vi "Control Panel.vi"(8 "error in (no error)":errorcluster, 11 "Fake Function Generator in":refnum<class "Function Generator.lvclass">) -> (0 "error out":errorcluster, 3 "Fake Function Generator out":refnum<class "Function Generator.lvclass">)   [LabVIEW 2009, in "Function Generator.lvclass"]
doc: "(Dynamic) A user-level application that simulates the physical front panel of the Instrument. Provide the user with buttons to manually control features of the instrument, and provide indicators of its current state."
uses:
  Function Generator.lvclass
  Tektronix AFG 3000 Series/controls.llb/Channel.ctl
  Tektronix AFG 3000 Series/controls.llb/Waveform Shape.ctl
  Tektronix AFG 3000 Series/controls.llb/Sweep Spacing.ctl
  Function Generator.lvclass/Function Generator.ctl
  Math Operations/To Start and Stop (bare).vi
  Math Operations/To Center and Span (frequency).vi
  Tektronix AFG 3000 Series/controls.llb/Voltage.ctl
  Tektronix AFG 3000 Series/controls.llb/Frequency Mode.ctl
  Tektronix AFG 3000 Series/controls.llb/Sweep Time Parameter.ctl
  Tektronix AFG 3000 Series/controls.llb/Sweep Frequency.ctl
  Math Operations/To Center and Span (bare).vi
  Math Operations/To Start and Stop (frequency).vi
  Tektronix AFG 3000 Series/Tektronix AFG 3000 Series.lvlib
  Utility Classes/Scannable/Scannable.lvclass
panel:
  in  "Ch2 on/off":bool
  in  "Ch1 on/off":bool
  out "Ready when blinking":bool
  in  "Set":bool
  in  "Read to control":bool
  in  "Read":bool
  in  "Copy actual to set":bool
  in  "Populate fields with member data":bool
  out "Start Freq.":dbl[unit]
  out "Stop Freq.":dbl[unit]
  out "Freq. Span":dbl[unit]
  out "Center Freq.":dbl[unit]
  out "Offset":dbl[unit]
  out "Amplitude":dbl[unit]
  out "High":dbl[unit]
  out "Low":dbl[unit]
  out "FM Source":u16(ring) items=["Internal", "External"]
  out "FM Modulation Waveform":u16(ring) items=["Sine", "Square", "Triangle", "Ramp", "Down Ramp", "Noise", "User 1", "User 2", "User 3", "User 4", "EMEMory", "EFILe"]
  out "FM Modulation Freq.":dbl[unit]=100.0
  out "FM Peak Deviation":dbl[unit]=100.0
  in  "FM Peak Deviation Set":dbl[unit]=100.0
  in  "FM Modulation Freq Set":dbl[unit]=100.0
  in  "FM Modulation Waveform Set":u16(ring) items=["Sine", "Square", "Triangle", "Ramp", "Down Ramp", "Noise", "User 1", "User 2", "User 3", "User 4", "EMEMory", "EFILe"]
  in  "FM Source Set":u16(ring) items=["Internal", "External"]
  out "AM Modulation Freq.":dbl[unit]=1000.0
  out "AM Modulation Waveform":u16(ring) items=["Sine", "Square", "Triangle", "Ramp", "Down Ramp", "Noise"]
  out "AM Source":u16(ring) items=["Internal", "External"]
  out "AM Modulation Depth":dbl
  in  "AM Modulation Depth Set":dbl
  in  "AM Modulation Freq. Set":dbl[unit]=1000.0
  in  "AM Modulation Waveform Set":u16(ring) items=["Sine", "Square", "Triangle", "Ramp", "Down Ramp", "Noise"]
  in  "AM Source Set":u16(ring) items=["Internal", "External"]
  out "Return Time":dbl[unit]
  out "Hold Time":dbl[unit]
  out "Sweep Time":dbl[unit]
  in  "Return Time Set":dbl[unit]
  in  "Hold Time Set":dbl[unit]
  in  "Sweep Time Set":dbl[unit] caption="Sweep time"
  out "Sweep Spacing":T1 items=["linear", "log"]
  in  "Sweep Spacing Set":T1 items=["linear", "log"]
  in  "Stop Freq. Set":dbl[unit]
  in  "Start Freq. Set":dbl[unit]
  out "Burst Mode":u16(ring)=1 items=["Triggered", "Gated"]
  out "Burst Count":i32=5
  in  "Burst Count Set":i32=5
  in  "Burst Mode Set":u16(ring)=1 items=["Triggered", "Gated"]
  out "Run Mode":u16(ring) items=["Continuous", "AM", "FM", "PM", "FSK", "PWM", "Sweep", "Burst"]
  in  "Run Mode Set":u16(ring) items=["Continuous", "AM", "FM", "PM", "FSK", "PWM", "Sweep", "Burst"]
  out "Trailing Edge Time":dbl[unit]
  out "Leading Edge Time":dbl[unit]
  out "Duty Cycle (%)":dbl
  in  "Duty Cycle Set (%)":dbl=50.0
  in  "Trailing Edge Time Set":dbl[unit]=5e-09 format="%#.6g"
  in  "Leading Edge Time Set":dbl[unit]=5e-09 format="%#.6g"
  out "Ramp Symm. (%)":dbl
  in  "Ramp Symm. Set (%)":dbl=50.0 min=0.0 max=100.0 step=1.0 format="%.2f"
  in  "Freq. Span Set":dbl[unit]
  in  "Center Freq. Set":dbl[unit]
  in  "Low Set":dbl[unit]
  in  "High Set":dbl[unit]
  in  "Amplitude Set":dbl[unit]
  in  "Offset Set":dbl[unit]
  in  "Exit":bool
  out "Waveform Shape":T2 items=["Sinusoid", "Square", "Pulse", "Ramp", "PRNoise", "DC", "SINC", "Gaussian", "Lorentz", "ERise", "EDecay", "Haversine", "User 1", "User 2", "User 3", "User 4", "EMemory", "EFile"]
  in  "Waveform Shape Set":T2 items=["Sinusoid", "Square", "Pulse", "Ramp", "PRNoise", "DC", "SINC", "Gaussian", "Lorentz", "ERise", "EDecay", "Haversine", "User 1", "User 2", "User 3", "User 4", "EMemory", "EFile"]
  out "Phase":dbl[unit]
  in  "Phase Set":dbl[unit]
  out "Frequency":dbl[unit]
  in  "Frequency Set":dbl[unit]
  in  "Channel":T3 items=["Channel 1", "Channel 2"]
  # "Tektronix AFG252 Function Generator Control Panel"
  # "VOLTAGE SETTINGS"
  # "SWEEP MODE SETTINGS"
  # "AM SETTINGS"
  # "GENERAL SETTINGS"
  # "RAMP SETTINGS"
  # "FM SETTINGS"
  # "Note: the program only sets\nthe values that are appropriate\nfor the run mode you select. I.e.,\nit won't set the FM settings if you\nselect \"Burst Mode\" here."
  # "PULSE SETTINGS"
  # "BURST MODE SETTINGS"
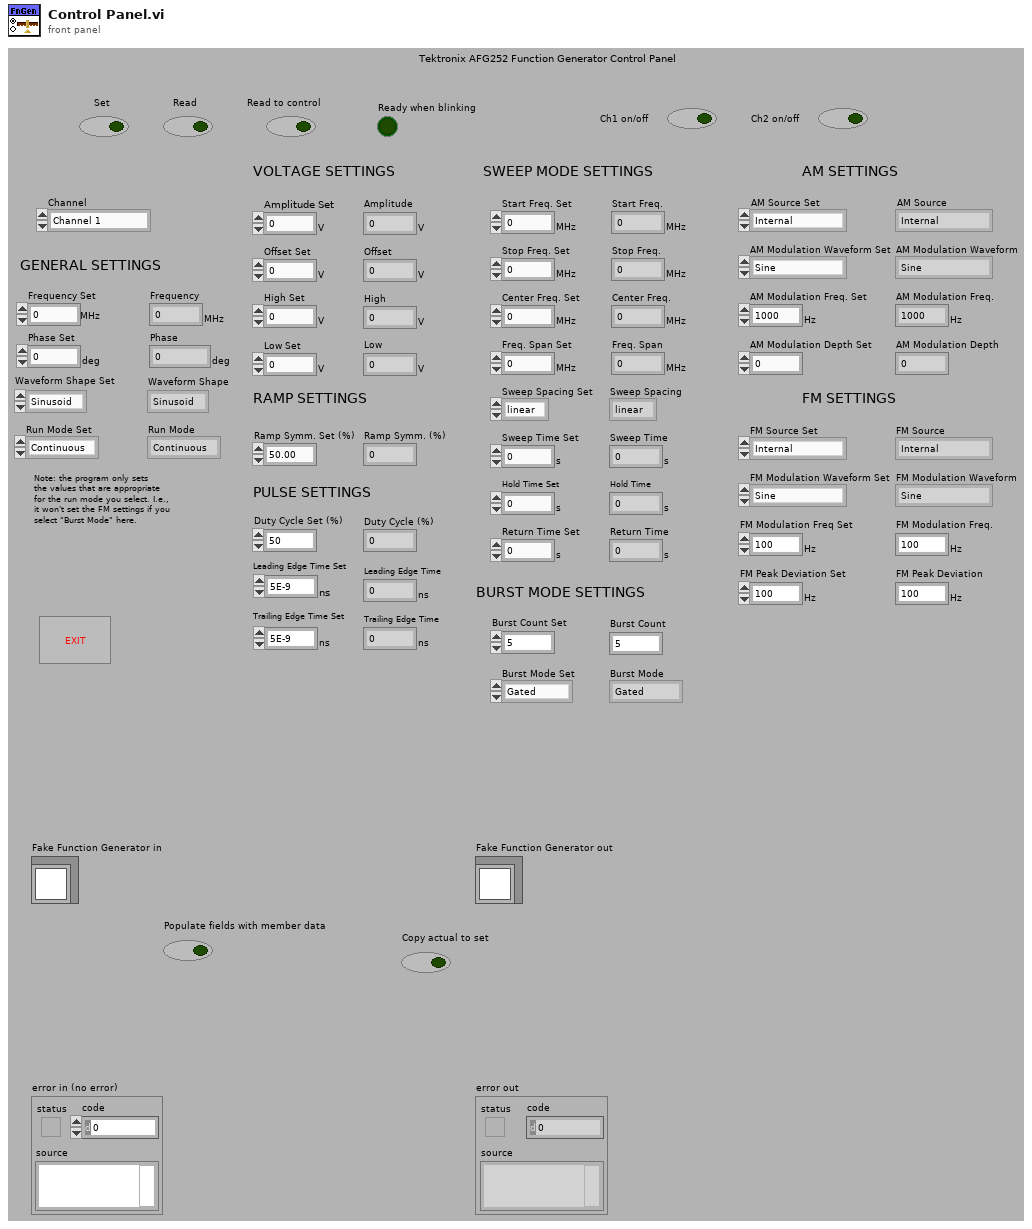
[diagram p1: front panel]
types:
  T1 = typedef "Sweep Spacing.ctl" = u16
  T2 = typedef "Waveform Shape.ctl" = u16
  T3 = typedef "Channel.ctl" = u16
  T4 = typedef "Voltage.ctl" = enum16{"amplitude", "offset", "high", "low", "high limit", "low limit"}
  T5 = typedef "Frequency Mode.ctl" = enum16{"CW", "Sweep"}
  T6 = typedef "Sweep Time Parameter.ctl" = enum16{"sweep time", "hold time", "return time"}
  T7 = typedef "Sweep Frequency.ctl" = enum16{"center", "span", "start", "stop"}
  T8 = typedef "FG Channel Settings.ctl" = cluster{"General Settings":cluster{" Frequency":dbl[unit], " Phase":dbl[unit], " Run Mode":u16, " Waveform Shape":T2, "Output on?":bool}, "Voltage Settings":cluster{"Amplitude":dbl[unit], "Offset":dbl[unit]}, "Ramp Settings":cluster{"Ramp Symmetry (%)":dbl}, "Pulse Settings":cluster{"Leading Edge Time ":dbl[unit], "Trailing Edge Time":dbl[unit], "Duty Cycle (%)":dbl}, "Sweep Mode Settings":cluster{"Start Freq. ":dbl[unit], "Stop Freq.  ":dbl[unit], "Sweep spacing":T1, "Sweep time":dbl[unit], "Hold time":dbl[unit], "Return time":dbl[unit]}, "Burst Mode Settings":cluster{"Burst Mode ":u16, "Burst Count":i32}, "AM Settings":cluster{"AM Source ":u16, "Modulation Waveform ":u16, "Modulation Frequency ":dbl[unit], "Modulation Depth ":dbl}, "FM Settings":cluster{"FM Source ":u16, "Modulation Waveform ":u16, "Modulation Frequency":dbl[unit], "Peak Deviation ":dbl[unit]}}
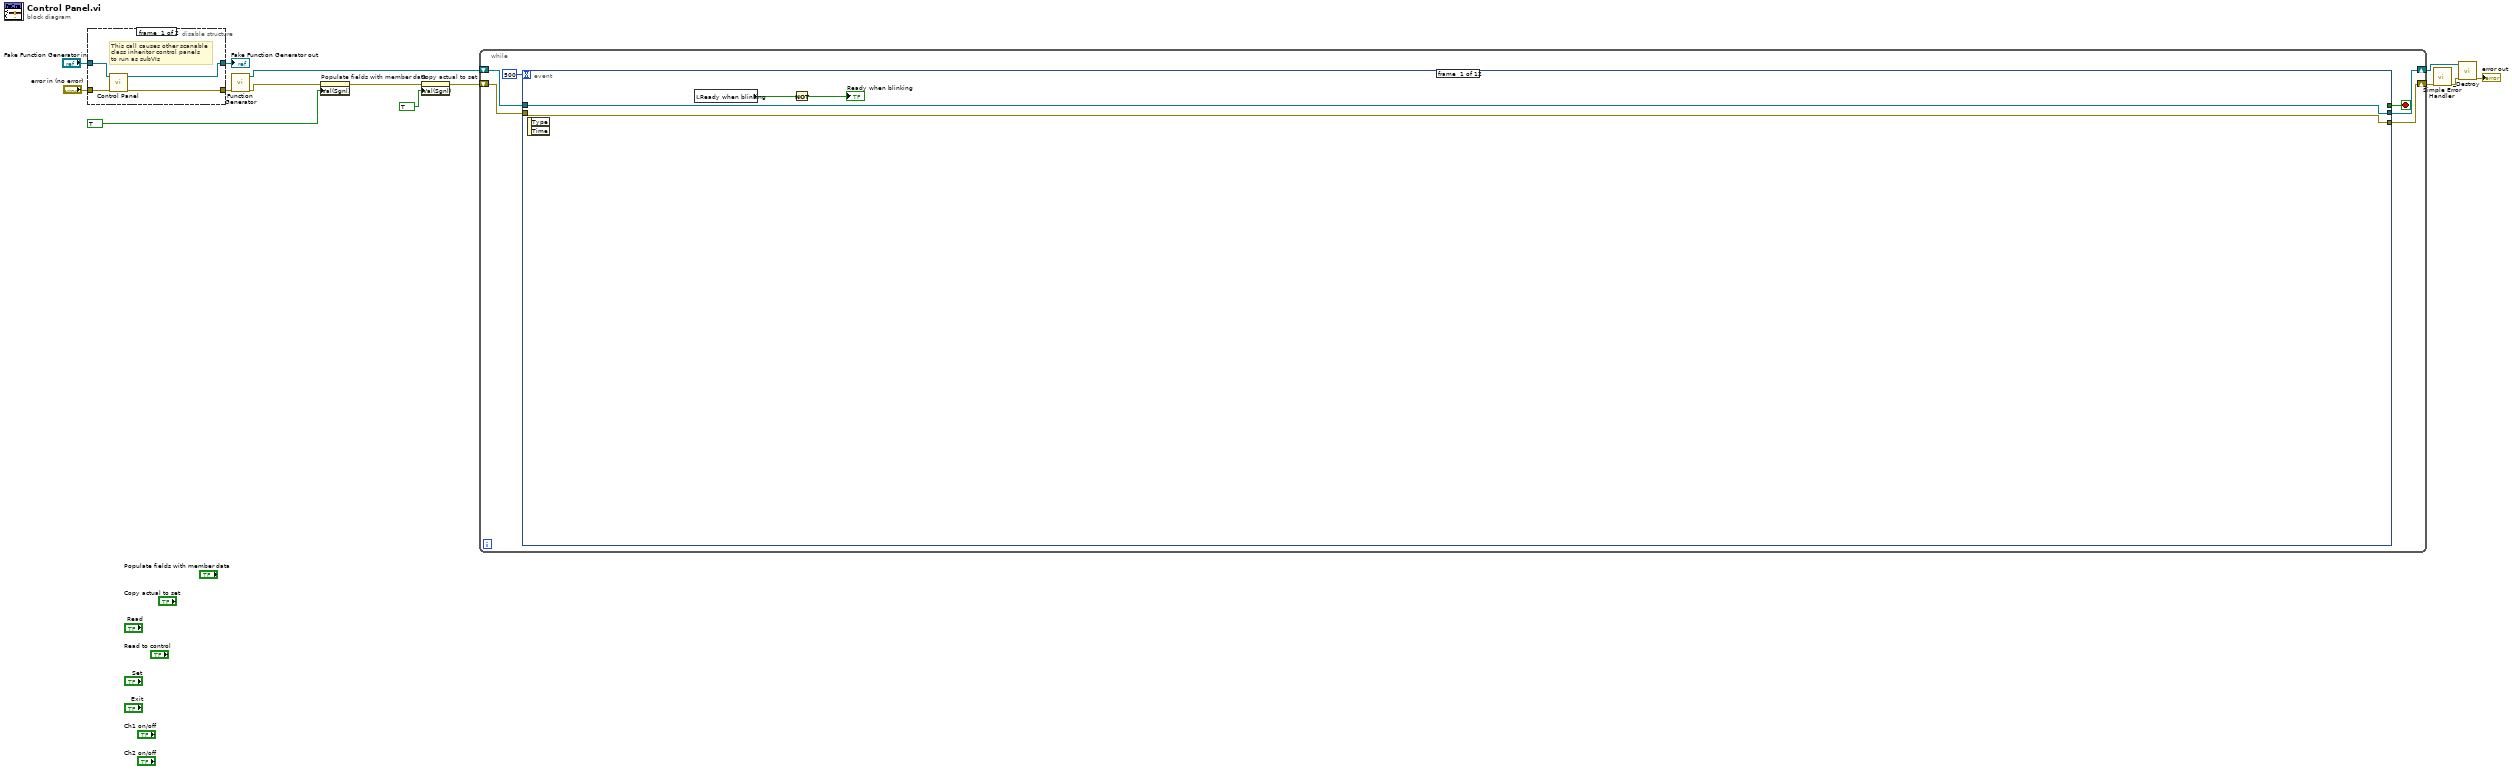
[diagram p0: block diagram]
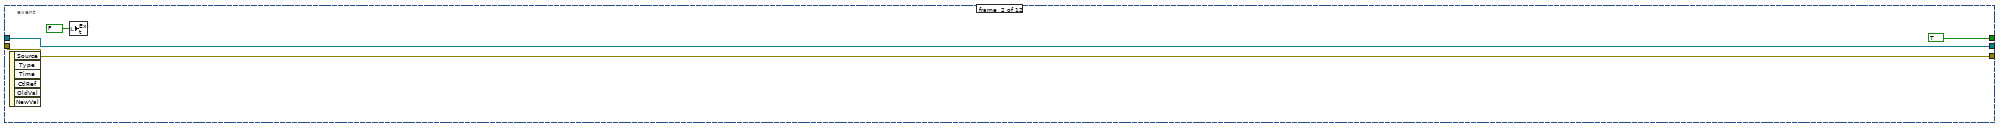
[diagram p3: hidden frame]
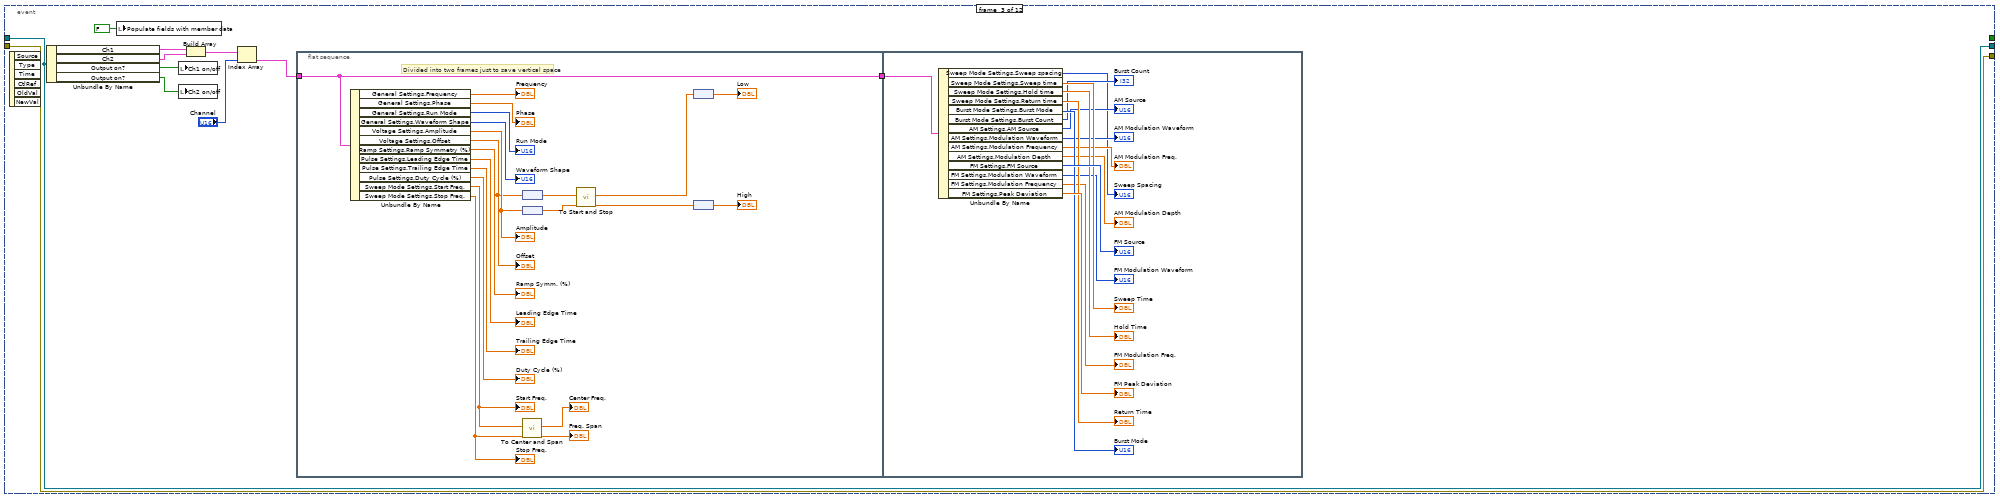
[diagram p4: hidden frame]
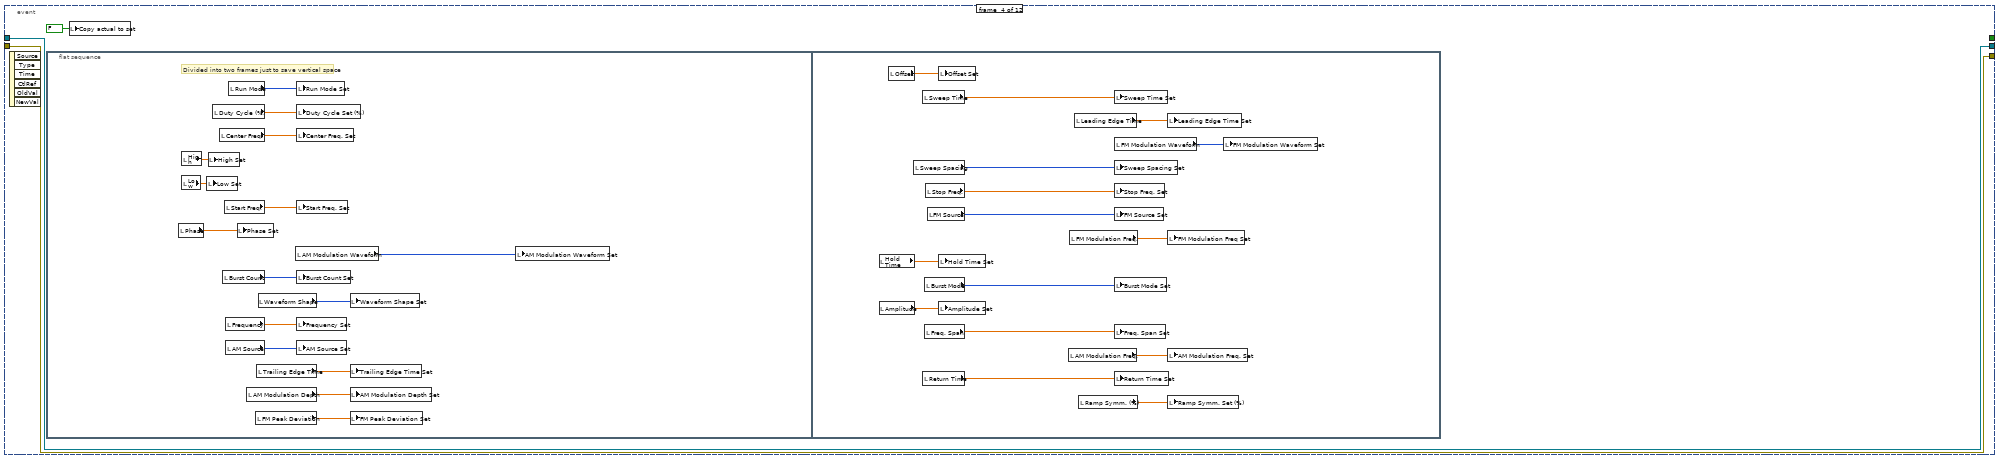
[diagram p5: hidden frame]
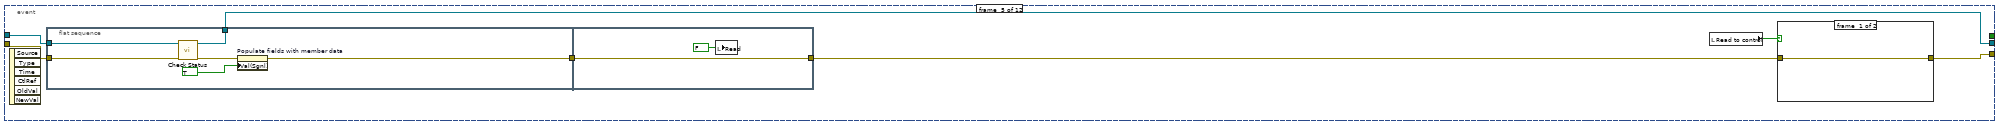
[diagram p6: hidden frame]
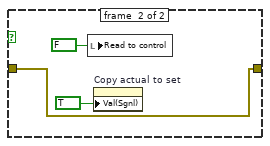
[diagram p7: hidden frame]
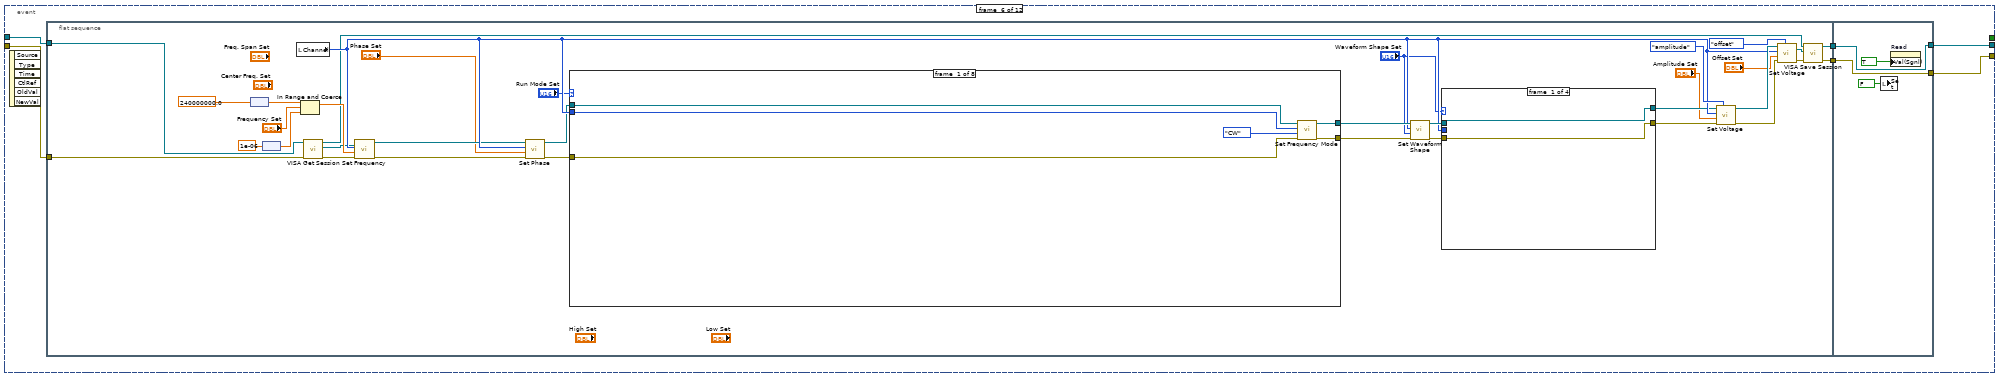
[diagram p8: hidden frame]
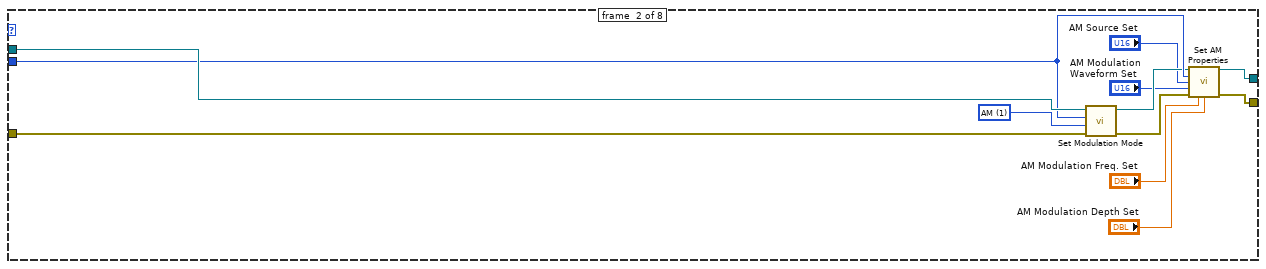
[diagram p9: hidden frame]
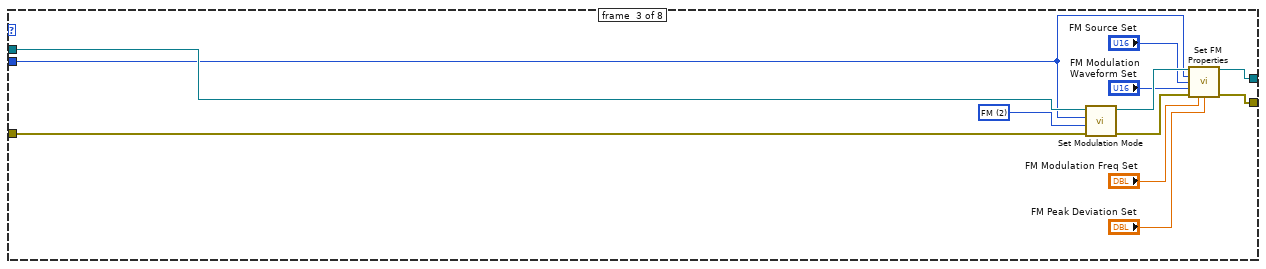
[diagram p10: hidden frame]
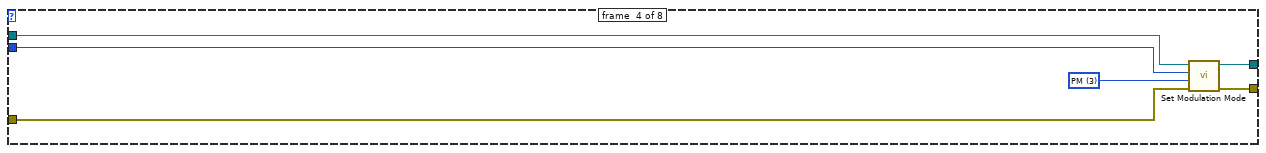
[diagram p11: hidden frame]
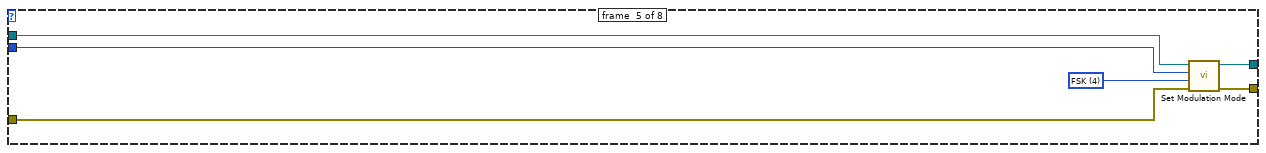
[diagram p12: hidden frame]
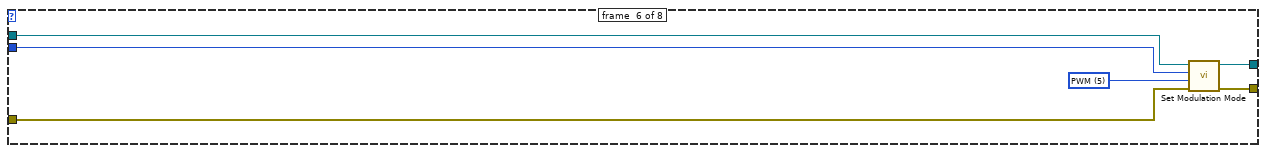
[diagram p13: hidden frame]
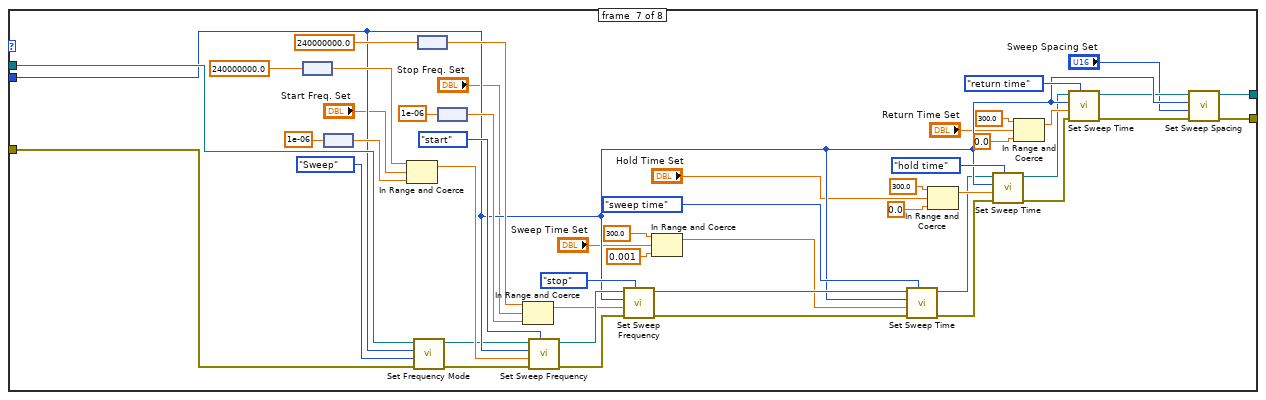
[diagram p14: hidden frame]
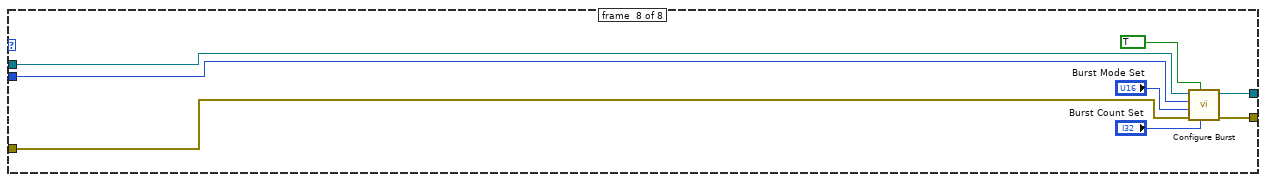
[diagram p15: hidden frame]
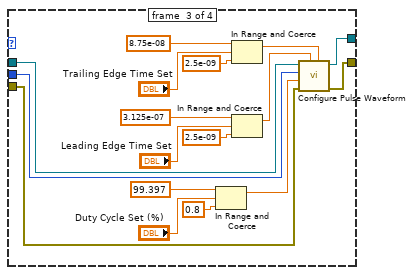
[diagram p17: hidden frame]
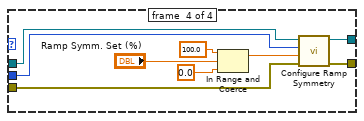
[diagram p18: hidden frame]
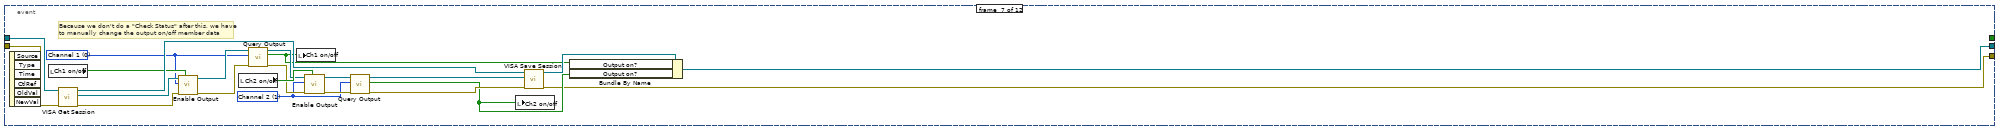
[diagram p19: hidden frame]
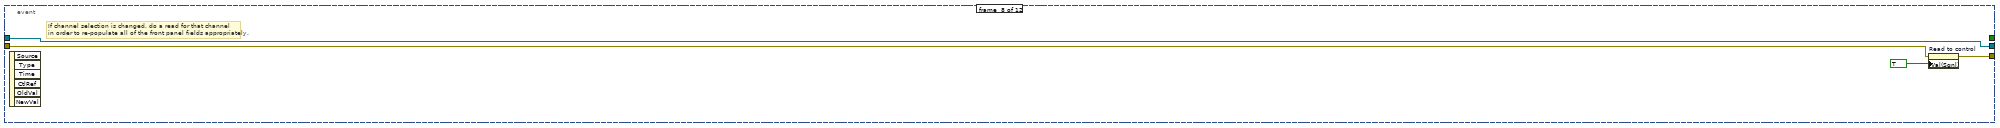
[diagram p20: hidden frame]
diagram:
  n1 = disable-structure shown="Enabled" {
    disable-tunnel: [w18 w20] -> w14
    disable-tunnel: "error in (no error)" -> [w17 w19]
    disable-tunnel: "Fake Function Generator in" -> [w16 w20]
    disable-tunnel: [w15 w19] -> w11
    frame #0 {
      # "This call causes other scanable\nclass inheritor control panels\nto run as subVIs"
      n2 = call-parent "Control Panel.vi"("error in (no error)"=w17, "Instrument in"=w16) -> ("error out"=w15:errorcluster, "Instrument out"=w18:refnum<class "Function Generator.lvclass">)  [unwired: 8 out]
    }
    frame #1 {
    }
  }
  "Fake Function Generator out" <- w14
  n3 = call "Function Generator.vi"("error in (no error)"=w11) -> ("error out"=w10:errorcluster, "Function Generator out"=w2:refnum<class "Function Generator.lvclass">)  [unwired: 9 out]
  n4 = property on="Populate fields with member data" class="Bool (strict)"(error in=w10, "Val(Sgnl)"=TRUE ("Value (Signaling)")) -> (error out=w7:errorcluster)  [unwired: 1 in, 1 out]
  n5 = property on="Copy actual to set" class="Bool (strict)"(error in=w7, "Val(Sgnl)"=TRUE ("Value (Signaling)")) -> (error out=w6:errorcluster)  [unwired: 1 in, 1 out]
  n6 = while {
    shift-right: [w26] -> w5
    shift-left: w6 -> [w25]
    shift-right: [w23] -> w1
    shift-left: w2 -> [w24]
    stop <- w21 stop-if-true
    n7 = event shown="[5] \"Set\": Value Change" {
      selector: _ -> [_ _ _ _ _ _ _ _ _ _ _ _]
      dyn-events: _ -> [_ _ _ _ _ _ _ _ _ _ _ _]
      timeout: 500 -> [_ _ _ _ _ _ _ _ _ _ _ _]
      tunnel: [w30 w31 w44 w83 w117 w136 w313 w336 w347 w357 w363 w369] -> w26
      tunnel: w25 -> [w30 w31 w44 w83 w118 w137 w325 w337 w347 w357 w363 w369]
      tunnel: [w29 w32 w43 w84 w115 w138 w316 w338 w348 w358 w364 w370] -> w23
      tunnel: w24 -> [w29 w32 w43 w84 w116 w139 w333 w338 w348 w358 w364 w370]
      tunnel: [_ TRUE ("Exit") _ _ _ _ _ _ _ _ _ _] -> w21
      event #0 {
        n8 = event-data() -> ()  [unwired: 3 out]
        n9 = local read "Ready when blinking"() -> (w28:bool)
        n10 = Not(x=w28) -> (.not. x?=→"Ready when blinking":bool)
      }
      event #1 {
        n11 = event-data() -> ()  [unwired: 7 out]
        n12 = local write "Exit"(FALSE ("Exit")) -> ()
      }
      event #2 {
        n13 = event-data() -> ()  [unwired: 7 out]
        n14 = Unbundle By Name(w43) -> ("Ch1"=w41:T8, "Ch2"=w42:T8, "Output on?"=w38:bool, "Output on?"=w37:bool)
        n15 = local write "Populate fields with member data"(FALSE ("Populate fields with member data")) -> ()
        n16 = local write "Ch1 on/off"(w38) -> ()
        n17 = local write "Ch2 on/off"(w37) -> ()
        n18 = Build Array(w41, w42) -> (w40:T8[])
        n19 = Index Array(array=w40, index="Channel") -> (element=w36:T8)
        n20 = flat-sequence {
          tunnel: w36 -> [w46]
          tunnel: [w46] -> w35
          tunnel: w35 -> [w67]
          frame #0 {
            # "Divided into two frames just to save vertical space"
            n21 = Unbundle By Name(w46) -> ("General Settings.Frequency"=→"Frequency":dbl[unit], "General Settings.Phase"=→"Phase":dbl[unit], "General Settings.Run Mode"=→"Run Mode":u16, "General Settings.Waveform Shape"=→"Waveform Shape":T2, "Voltage Settings.Amplitude"=w54:dbl[unit], "Voltage Settings.Offset"=w53:dbl[unit], "Ramp Settings.Ramp Symmetry (%)"=→"Ramp Symm. (%)":dbl, "Pulse Settings.Leading Edge Time"=→"Leading Edge Time":dbl[unit], "Pulse Settings.Trailing Edge Time"=→"Trailing Edge Time":dbl[unit], "Pulse Settings.Duty Cycle (%)"=→"Duty Cycle (%)":dbl, "Sweep Mode Settings.Start Freq."=w48:dbl[unit], "Sweep Mode Settings.Stop Freq."=w47:dbl[unit])
            "Amplitude" <- w54
            "Offset" <- w53
            "Stop Freq." <- w47
            "Start Freq." <- w48
            n22 = node(w53) -> (w63:dbl)
            n23 = node(w54) -> (w64:dbl)
            n24 = call-poly "To Center and Span.vi"("stop"=w47, "start"=w48) -> ("span"=→"Freq. Span":dbl[unit], "center"=→"Center Freq.":dbl[unit])  [unwired: 4 out]
            n25 = call-poly "To Start and Stop.vi"("span"=w64, "center"=w63) -> ("stop"=w61:dbl, "start"=w62:dbl)  [unwired: 4 out]
            n26 = node(w62) -> (→"Low":dbl[unit])
            n27 = node(w61) -> (→"High":dbl[unit])
          }
          frame #1 {
            n28 = Unbundle By Name(w67) -> ("Sweep Mode Settings.Sweep spacing"=→"Sweep Spacing":T1, "Sweep Mode Settings.Sweep time"=→"Sweep Time":dbl[unit], "Sweep Mode Settings.Hold time"=→"Hold Time":dbl[unit], "Sweep Mode Settings.Return time"=→"Return Time":dbl[unit], "Burst Mode Settings.Burst Mode"=→"Burst Mode":u16, "Burst Mode Settings.Burst Count"=→"Burst Count":i32, "AM Settings.AM Source"=→"AM Source":u16, "AM Settings.Modulation Waveform"=→"AM Modulation Waveform":u16, "AM Settings.Modulation Frequency"=→"AM Modulation Freq.":dbl[unit], "AM Settings.Modulation Depth"=→"AM Modulation Depth":dbl, "FM Settings.FM Source"=→"FM Source":u16, "FM Settings.Modulation Waveform"=→"FM Modulation Waveform":u16, "FM Settings.Modulation Frequency"=→"FM Modulation Freq.":dbl[unit], "FM Settings.Peak Deviation"=→"FM Peak Deviation":dbl[unit])
          }
        }
      }
      event #3 {
        n29 = event-data() -> ()  [unwired: 7 out]
        n30 = flat-sequence {
          frame #0 {
            # "Divided into two frames just to save vertical space"
            n31 = local read "Phase"() -> (w96:dbl[unit])
            n32 = local read "High"() -> (w95:dbl[unit])
            n33 = local read "Low"() -> (w94:dbl[unit])
            n34 = local write "Low Set"(w94) -> ()
            n35 = local write "High Set"(w95) -> ()
            n36 = local read "Duty Cycle (%)"() -> (w93:dbl)
            n37 = local read "Center Freq."() -> (w90:dbl[unit])
            n38 = local read "Burst Count"() -> (w89:i32)
            n39 = local read "Start Freq."() -> (w91:dbl[unit])
            n40 = local read "Frequency"() -> (w99:dbl[unit])
            n41 = local read "AM Source"() -> (w88:u16)
            n42 = local read "Run Mode"() -> (w97:u16)
            n43 = local write "Phase Set"(w96) -> ()
            n44 = local read "AM Modulation Depth"() -> (w86:dbl)
            n45 = local read "FM Peak Deviation"() -> (w85:dbl[unit])
            n46 = local read "Trailing Edge Time"() -> (w92:dbl[unit])
            n47 = local read "Waveform Shape"() -> (w98:T2)
            n48 = local read "AM Modulation Waveform"() -> (w87:u16)
            n49 = local write "Run Mode Set"(w97) -> ()
            n50 = local write "Duty Cycle Set (%)"(w93) -> ()
            n51 = local write "Center Freq. Set"(w90) -> ()
            n52 = local write "Start Freq. Set"(w91) -> ()
            n53 = local write "Burst Count Set"(w89) -> ()
            n54 = local write "Frequency Set"(w99) -> ()
            n55 = local write "AM Source Set"(w88) -> ()
            n56 = local write "Waveform Shape Set"(w98) -> ()
            n57 = local write "Trailing Edge Time Set"(w92) -> ()
            n58 = local write "AM Modulation Depth Set"(w86) -> ()
            n59 = local write "FM Peak Deviation Set"(w85) -> ()
            n60 = local write "AM Modulation Waveform Set"(w87) -> ()
          }
          frame #1 {
            n61 = local read "Hold Time"() -> (w108:dbl[unit])
            n62 = local read "Amplitude"() -> (w100:dbl[unit])
            n63 = local read "Offset"() -> (w101:dbl[unit])
            n64 = local read "Sweep Spacing"() -> (w106:T1)
            n65 = local read "Sweep Time"() -> (w107:dbl[unit])
            n66 = local read "Return Time"() -> (w109:dbl[unit])
            n67 = local read "Burst Mode"() -> (w110:u16)
            n68 = local read "Freq. Span"() -> (w105:dbl[unit])
            n69 = local read "Stop Freq."() -> (w104:dbl[unit])
            n70 = local read "FM Source"() -> (w112:u16)
            n71 = local write "Offset Set"(w101) -> ()
            n72 = local write "Hold Time Set"(w108) -> ()
            n73 = local write "Amplitude Set"(w100) -> ()
            n74 = local read "AM Modulation Freq."() -> (w111:dbl[unit])
            n75 = local read "FM Modulation Freq."() -> (w114:dbl[unit])
            n76 = local read "Leading Edge Time"() -> (w103:dbl[unit])
            n77 = local read "Ramp Symm. (%)"() -> (w102:dbl)
            n78 = local write "Sweep Time Set"(w107) -> ()
            n79 = local write "Sweep Spacing Set"(w106) -> ()
            n80 = local write "Stop Freq. Set"(w104) -> ()
            n81 = local write "FM Source Set"(w112) -> ()
            n82 = local write "Burst Mode Set"(w110) -> ()
            n83 = local write "Freq. Span Set"(w105) -> ()
            n84 = local write "Return Time Set"(w109) -> ()
            n85 = local read "FM Modulation Waveform"() -> (w113:u16)
            n86 = local write "Leading Edge Time Set"(w103) -> ()
            n87 = local write "FM Modulation Freq Set"(w114) -> ()
            n88 = local write "AM Modulation Freq. Set"(w111) -> ()
            n89 = local write "Ramp Symm. Set (%)"(w102) -> ()
            n90 = local write "FM Modulation Waveform Set"(w113) -> ()
          }
        }
        n91 = local write "Copy actual to set"(FALSE ("Copy actual to set")) -> ()
      }
      event #4 {
        n92 = event-data() -> ()  [unwired: 7 out]
        n93 = flat-sequence {
          tunnel: [w126] -> w119
          tunnel: w118 -> [w128]
          tunnel: w116 -> [w131]
          tunnel: [w130] -> w115
          tunnel: [w133] -> w120
          tunnel: w119 -> [w133]
          frame #0 {
            n94 = call-dynamic "Check Status.vi"("error in (no error)"=w128, "Function Generator in"=w131) -> ("error out"=w127:errorcluster, "Function Generator out"=w130:refnum<class "Function Generator.lvclass">)  [unwired: 8 out]
            n95 = property on="Populate fields with member data" class="Bool (strict)"(error in=w127, "Val(Sgnl)"=TRUE ("Value (Signaling)")) -> (error out=w126:errorcluster)  [unwired: 1 in, 1 out]
          }
          frame #1 {
            n96 = local write "Read"(FALSE ("Read")) -> ()
          }
        }
        n97 = local read "Read to control"() -> (w121:bool)
        n98 = case shown="True" w121 {
          tunnel: [w122 w124] -> w117
          tunnel: w120 -> [w122 w124]
          frame #0 {
          }
          frame #1 {
            n99 = local write "Read to control"(FALSE ("Read")) -> ()
            n100 = property on="Copy actual to set" class="Bool (strict)"("Val(Sgnl)"=TRUE ("Value (Signaling)")) -> ()  [unwired: 2 in, 2 out]
          }
        }
      }
      event #5 {
        n101 = event-data() -> ()  [unwired: 7 out]
        n102 = flat-sequence {
          tunnel: w139 -> [w159]
          tunnel: w137 -> [w157]
          tunnel: [w158] -> w135
          tunnel: [w142] -> w134
          tunnel: [w311] -> w136
          tunnel: [w312] -> w138
          tunnel: w135 -> [w312]
          tunnel: w134 -> [w311]
          frame #0 {
            n103 = node(240000000.0 ("upper limit")) -> (w171:dbl[unit])
            n104 = node(1e-06 ("lower limit")) -> (w172:dbl[unit])
            n105 = local read "Channel"() -> (w161:T3)
            n106 = In Range and Coerce(upper limit=w171, x="Frequency Set", lower limit=w172) -> (coerced(x)=w166:dbl[unit])  [unwired: 1 out]
            n107 = call-dynamic "VISA Get Session.vi"("error in (no error)"=w157, "Instrument.lvclass in"=w159) -> ("error out"=w156:errorcluster, "VISA Resource Name"=w155:refnum<visa-resource-name>, "Instrument.lvclass out"=w160:refnum<class "Function Generator.lvclass">)  [unwired: 7 out]
            n108 = call "Set Frequency.vi"("error in (no error)"=w156, "frequency"=w166, "Channel (0: Channel 1)"=w161, "VISA resource name"=w155) -> ("error out"=w153:errorcluster, "VISA resource name out"=w154:refnum<visa-resource-name>)  [unwired: 6 out]
            n109 = call "Set Phase.vi"("error in (no error)"=w153, "phase"="Phase Set", "Channel (0: Channel 1)"=w161, "VISA resource name"=w154) -> ("error out"=w151:errorcluster, "VISA resource name out"=w152:refnum<visa-resource-name>)  [unwired: 1 in, 5 out]
            n110 = case shown="1" "Run Mode Set" {
              tunnel: w152 -> [w179 w191 w204 w209 w215 w222 w270 w278]
              tunnel: w151 -> [w178 w190 w203 w208 w214 w221 w269 w277]
              tunnel: w161 -> [w177 w189 w199 w207 w213 w220 w240 w276]
              tunnel: [w176 w182 w194 w206 w212 w218 w232 w274] -> w163
              tunnel: [w175 w181 w193 w205 w211 w217 w231 w273] -> w162
              frame #0 {
                n111 = call "Set Frequency Mode.vi"("error in (no error)"=w178, "Mode (0: CW)"=Frequency_Mode."CW", "Channel (0: Channel 1)"=w177, "VISA resource name"=w179) -> ("error out"=w175:errorcluster, "VISA resource name out"=w176:refnum<visa-resource-name>)  [unwired: 6 out]
              }
              frame #1 {
                w192 = u16 1 items=["n/a", "AM", "FM", "PM", "FSK", "PWM"] ("Modulation Mode (def: AM)")
                n112 = call "Set Modulation Mode.vi"("error in (no error)"=w190, "Modulation Mode (def: AM)"=w192, "Channel (0: Channel 1)"=w189, "VISA resource name"=w191) -> ("error out"=w187:errorcluster, "VISA resource name out"=w188:refnum<visa-resource-name>)  [unwired: 6 out]
                n113 = call "Set AM Properties.vi"("VISA resource name"=w188, "Channel (0: Channel 1)"=w189, "AM Source (0: Internal)"="AM Source Set", "Modulation Waveform (0: Sine)"="AM Modulation Waveform Set", "error in (no error)"=w187, "Modulation Frequency (1000 Hz)"="AM Modulation Freq. Set", "Modulation Depth (0 %)"="AM Modulation Depth Set") -> ("VISA resource name out"=w182:refnum<visa-resource-name>, "error out"=w181:errorcluster)  [unwired: 7 out]
              }
              frame #2 {
                w202 = u16 2 items=["n/a", "AM", "FM", "PM", "FSK", "PWM"] ("Modulation Mode (def: AM)")
                n114 = call "Set Modulation Mode.vi"("error in (no error)"=w203, "Modulation Mode (def: AM)"=w202, "Channel (0: Channel 1)"=w199, "VISA resource name"=w204) -> ("error out"=w201:errorcluster, "VISA resource name out"=w200:refnum<visa-resource-name>)  [unwired: 6 out]
                n115 = call "Set FM Properties.vi"("VISA resource name"=w200, "Channel (0: Channel 1)"=w199, "FM Source (0: Internal)"="FM Source Set", "Modulation Waveform (0: Sine)"="FM Modulation Waveform Set", "error in (no error)"=w201, "Modulation Frequency (100.00 Hz)"="FM Modulation Freq Set", "Peak Deviation (100.00 Hz)"="FM Peak Deviation Set") -> ("VISA resource name out"=w194:refnum<visa-resource-name>, "error out"=w193:errorcluster)  [unwired: 7 out]
              }
              frame #3 {
                w210 = u16 3 items=["n/a", "AM", "FM", "PM", "FSK", "PWM"] ("Modulation Mode (def: AM)")
                n116 = call "Set Modulation Mode.vi"("error in (no error)"=w208, "Modulation Mode (def: AM)"=w210, "Channel (0: Channel 1)"=w207, "VISA resource name"=w209) -> ("error out"=w205:errorcluster, "VISA resource name out"=w206:refnum<visa-resource-name>)  [unwired: 6 out]
              }
              frame #4 {
                w216 = u16 4 items=["n/a", "AM", "FM", "PM", "FSK", "PWM"] ("Modulation Mode (def: AM)")
                n117 = call "Set Modulation Mode.vi"("error in (no error)"=w214, "Modulation Mode (def: AM)"=w216, "Channel (0: Channel 1)"=w213, "VISA resource name"=w215) -> ("error out"=w211:errorcluster, "VISA resource name out"=w212:refnum<visa-resource-name>)  [unwired: 6 out]
              }
              frame #5 {
                w219 = u16 5 items=["n/a", "AM", "FM", "PM", "FSK", "PWM"] ("Modulation Mode (def: AM)")
                n118 = call "Set Modulation Mode.vi"("error in (no error)"=w221, "Modulation Mode (def: AM)"=w219, "Channel (0: Channel 1)"=w220, "VISA resource name"=w222) -> ("error out"=w217:errorcluster, "VISA resource name out"=w218:refnum<visa-resource-name>)  [unwired: 6 out]
              }
              frame #6 {
                n119 = node(240000000.0 ("upper limit")) -> (w263:dbl[unit])
                n120 = node(1e-06 ("lower limit")) -> (w264:dbl[unit])
                n121 = In Range and Coerce(upper limit=w263, x="Start Freq. Set", lower limit=w264) -> (coerced(x)=w241:dbl[unit])  [unwired: 1 out]
                n122 = call "Set Frequency Mode.vi"("error in (no error)"=w269, "Mode (0: CW)"=Frequency_Mode."Sweep", "Channel (0: Channel 1)"=w240, "VISA resource name"=w270) -> ("error out"=w223:errorcluster, "VISA resource name out"=w224:refnum<visa-resource-name>)  [unwired: 6 out]
                n123 = node(240000000.0 ("upper limit")) -> (w260:dbl[unit])
                n124 = node(1e-06 ("lower limit")) -> (w261:dbl[unit])
                n125 = In Range and Coerce(upper limit=w260, x="Stop Freq. Set", lower limit=w261) -> (coerced(x)=w257:dbl[unit])  [unwired: 1 out]
                n126 = call "Set Sweep Frequency.vi"("Sweep Frequency"=Sweep_Frequency."start", "error in (no error)"=w223, "frequency"=w241, "Channel (0: Channel 1)"=w240, "VISA resource name"=w224) -> ("error out"=w258:errorcluster, "VISA resource name out"=w259:refnum<visa-resource-name>)  [unwired: 5 out]
                n127 = call "Set Sweep Frequency.vi"("Sweep Frequency"=Sweep_Frequency."stop", "error in (no error)"=w258, "frequency"=w257, "Channel (0: Channel 1)"=w240, "VISA resource name"=w259) -> ("error out"=w252:errorcluster, "VISA resource name out"=w253:refnum<visa-resource-name>)  [unwired: 5 out]
                n128 = In Range and Coerce(upper limit=dbl[unit] 300.0, x="Sweep Time Set", lower limit=dbl[unit] 0.001) -> (coerced(x)=w247:dbl[unit])  [unwired: 1 out]
                n129 = call "Set Sweep Time.vi"("Sweep Time Param (sweep time)"=Sweep_Time_Parameter."sweep time", "error in (no error)"=w252, "time"=w247, "Channel (0: Channel 1)"=w240, "VISA resource name"=w253) -> ("error out"=w237:errorcluster, "VISA resource name out"=w238:refnum<visa-resource-name>)  [unwired: 5 out]
                n130 = In Range and Coerce(upper limit=dbl[unit] 300.0, x="Hold Time Set", lower limit=dbl[unit] 0.0) -> (coerced(x)=w244:dbl[unit])  [unwired: 1 out]
                n131 = call "Set Sweep Time.vi"("Sweep Time Param (sweep time)"=Sweep_Time_Parameter."hold time", "error in (no error)"=w237, "time"=w244, "Channel (0: Channel 1)"=w240, "VISA resource name"=w238) -> ("error out"=w235:errorcluster, "VISA resource name out"=w236:refnum<visa-resource-name>)  [unwired: 5 out]
                n132 = In Range and Coerce(upper limit=dbl[unit] 300.0, x="Return Time Set", lower limit=dbl[unit] 0.0) -> (coerced(x)=w243:dbl[unit])  [unwired: 1 out]
                n133 = call "Set Sweep Time.vi"("Sweep Time Param (sweep time)"=Sweep_Time_Parameter."return time", "error in (no error)"=w235, "time"=w243, "Channel (0: Channel 1)"=w240, "VISA resource name"=w236) -> ("error out"=w233:errorcluster, "VISA resource name out"=w234:refnum<visa-resource-name>)  [unwired: 5 out]
                n134 = call "Set Sweep Spacing.vi"("error in (no error)"=w233, "Sweep spacing (linear)"="Sweep Spacing Set", "Channel (0: Channel 1)"=w240, "VISA resource name"=w234) -> ("error out"=w231:errorcluster, "VISA resource name out"=w232:refnum<visa-resource-name>)  [unwired: 6 out]
              }
              frame #7 {
                n135 = call "Configure Burst.vi"("Burst Count (5)"="Burst Count Set", "Enable Burst (T: Enable)"=TRUE, "error in (no error)"=w277, "Burst Mode (0: Triggered)"="Burst Mode Set", "Channel (0: Channel 1)"=w276, "VISA resource name"=w278) -> ("error out"=w273:errorcluster, "VISA resource name out"=w274:refnum<visa-resource-name>)  [unwired: 4 out]
              }
            }
            n136 = call "Set Waveform Shape.vi"("error in (no error)"=w162, "Waveform Shape"="Waveform Shape Set", "Channel (0: Channel 1)"=w161, "VISA resource name"=w163) -> ("error out"=w164:errorcluster, "VISA resource name out"=w165:refnum<visa-resource-name>)  [unwired: 6 out]
            n137 = case shown="0, Default" "Waveform Shape Set" {
              tunnel: w165 -> [w280 w282 w299 w308]
              tunnel: w164 -> [w279 w281 w298 w307]
              tunnel: [w280 w282 w284 w301] -> w148
              tunnel: [w279 w281 w283 w300] -> w147
              tunnel: w161 -> [_ _ w288 w303]
              frame #0 {
              }
              frame #1 {
              }
              frame #2 {
                n138 = In Range and Coerce(upper limit=99.397, x="Duty Cycle Set (%)", lower limit=0.8) -> (coerced(x)=w289:dbl)  [unwired: 1 out]
                n139 = In Range and Coerce(upper limit=dbl[unit] 8.75e-08, x="Trailing Edge Time Set", lower limit=dbl[unit] 2.5e-09) -> (coerced(x)=w292:dbl[unit])  [unwired: 1 out]
                n140 = In Range and Coerce(upper limit=dbl[unit] 3.125e-07, x="Leading Edge Time Set", lower limit=dbl[unit] 2.5e-09) -> (coerced(x)=w295:dbl[unit])  [unwired: 1 out]
                n141 = call "Configure Pulse Waveform.vi"("Trailing Edge Time (5.0E-9 s)"=w292, "Leading Edge Time (5.0E-9 s)"=w295, "error in (no error)"=w298, "Duty Cycle (50%)"=w289, "Channel (0: Channel 1)"=w288, "VISA resource name"=w299) -> ("error out"=w283:errorcluster, "VISA resource name out"=w284:refnum<visa-resource-name>)  [unwired: 1 in, 3 out]
              }
              frame #3 {
                n142 = In Range and Coerce(upper limit=100.0, x="Ramp Symm. Set (%)", lower limit=0.0) -> (coerced(x)=w304:dbl)  [unwired: 1 out]
                n143 = call "Configure Ramp Symmetry.vi"("error in (no error)"=w307, "Ramp Symmetry (50.00 %)"=w304, "Channel (0: Channel 1)"=w303, "VISA resource name"=w308) -> ("error out"=w300:errorcluster, "VISA resource name out"=w301:refnum<visa-resource-name>)  [unwired: 6 out]
              }
            }
            n144 = call "Set Voltage.vi"("Voltage Param (amplitude)"=Voltage."amplitude", "error in (no error)"=w147, "voltage"="Amplitude Set", "Channel (0: Channel 1)"=w161, "VISA resource name"=w148) -> ("error out"=w169:errorcluster, "VISA resource name out"=w168:refnum<visa-resource-name>)  [unwired: 5 out]
            n145 = call "Set Voltage.vi"("Voltage Param (amplitude)"=Voltage."offset", "error in (no error)"=w169, "voltage"="Offset Set", "Channel (0: Channel 1)"=w161, "VISA resource name"=w168) -> ("error out"=w143:errorcluster, "VISA resource name out"=w144:refnum<visa-resource-name>)  [unwired: 5 out]
            n146 = call-dynamic "VISA Save Session.vi"("error in (no error)"=w143, "VISA Resource Name"=w144, "Instrument.lvclass in"=w160) -> ("error out"=w142:errorcluster, "Instrument.lvclass out"=w158:refnum<class "Function Generator.lvclass">)  [unwired: 7 out]
          }
          frame #1 {
            n147 = local write "Set"(FALSE ("Set")) -> ()
            n148 = property on="Read" class="Bool (strict)"("Val(Sgnl)"=TRUE ("Value (Signaling)")) -> ()  [unwired: 2 in, 2 out]
          }
        }
      }
      event #6 {
        w318 = T3 1 items=["Channel 1", "Channel 2"] ("Channel (0: Channel 1)")
        w319 = T3 0 items=["Channel 1", "Channel 2"] ("Channel (0: Channel 1)")
        # "Because we don't do a \"Check Status\" after this, we have \nto manually change the output on/off member data"
        n149 = event-data() -> ()  [unwired: 7 out]
        n150 = local read "Ch1 on/off"() -> (w332:bool)
        n151 = call-dynamic "VISA Get Session.vi"("error in (no error)"=w325, "Instrument.lvclass in"=w333) -> ("error out"=w324:errorcluster, "VISA Resource Name"=w330:refnum<visa-resource-name>, "Instrument.lvclass out"=w334:refnum<class "Function Generator.lvclass">)  [unwired: 7 out]
        n152 = call "Enable Output.vi"("Enable Output (T: Enable)"=w332, "error in (no error)"=w324, "Channel (0: Channel 1)"=w319, "VISA resource name"=w330) -> ("error out"=w323:errorcluster, "VISA resource name out"=w329:refnum<visa-resource-name>)  [unwired: 6 out]
        n153 = local read "Ch2 on/off"() -> (w331:bool)
        n154 = call "Query Output.vi"("error in (no error)"=w323, "Channel (0: Channel 1)"=w319, "VISA resource name"=w329) -> ("error out"=w322:errorcluster, "Output Enabled?"=w315:bool, "VISA resource name out"=w328:refnum<visa-resource-name>)  [unwired: 6 out]
        n155 = local write "Ch1 on/off"(w315) -> ()
        n156 = call "Enable Output.vi"("Enable Output (T: Enable)"=w331, "error in (no error)"=w322, "Channel (0: Channel 1)"=w318, "VISA resource name"=w328) -> ("error out"=w321:errorcluster, "VISA resource name out"=w327:refnum<visa-resource-name>)  [unwired: 6 out]
        n157 = call "Query Output.vi"("error in (no error)"=w321, "Channel (0: Channel 1)"=w318, "VISA resource name"=w327) -> ("error out"=w320:errorcluster, "Output Enabled?"=w314:bool, "VISA resource name out"=w326:refnum<visa-resource-name>)  [unwired: 6 out]
        n158 = local write "Ch2 on/off"(w314) -> ()
        n159 = call-dynamic "VISA Save Session.vi"("error in (no error)"=w320, "VISA Resource Name"=w326, "Instrument.lvclass in"=w334) -> ("error out"=w313:errorcluster, "Instrument.lvclass out"=w317:refnum<class "Function Generator.lvclass">)  [unwired: 7 out]
        n160 = Bundle By Name(cluster=w317, "Output on?"=w315, "Output on?"=w314) -> (w316:refnum<class "Function Generator.lvclass">)
      }
      event #7 {
        # "If channel selection is changed, do a read for that channel\nin order to re-populate all of the front panel fields appropriately."
        n161 = event-data() -> ()  [unwired: 7 out]
        n162 = property on="Read to control" class="Bool (strict)"(error in=w337, "Val(Sgnl)"=TRUE ("Value (Signaling)")) -> (error out=w336:errorcluster)  [unwired: 1 in, 1 out]
      }
      event #8 {
        n163 = event-data() -> ()  [unwired: 7 out]
        n164 = local read "Amplitude Set"() -> (w341:dbl[unit])
        n165 = local read "Offset Set"() -> (w342:dbl[unit])
        n166 = node(w342) -> (w344:dbl)
        n167 = node(w341) -> (w343:dbl)
        n168 = call-poly "To Start and Stop.vi"("span"=w343, "center"=w344) -> ("stop"=w346:dbl, "start"=w345:dbl)  [unwired: 4 out]
        n169 = node(w345) -> (w340:dbl[unit])
        n170 = node(w346) -> (w339:dbl[unit])
        n171 = local write "Low Set"(w340) -> ()
        n172 = local write "High Set"(w339) -> ()
      }
      event #9 {
        n173 = event-data() -> ()  [unwired: 7 out]
        n174 = local read "High Set"() -> (w352:dbl[unit])
        n175 = local read "Low Set"() -> (w351:dbl[unit])
        n176 = node(w351) -> (w356:dbl)
        n177 = node(w352) -> (w355:dbl)
        n178 = call-poly "To Center and Span.vi"("stop"=w355, "start"=w356) -> ("span"=w353:dbl, "center"=w354:dbl)  [unwired: 4 out]
        n179 = node(w354) -> (w350:dbl[unit])
        n180 = node(w353) -> (w349:dbl[unit])
        n181 = local write "Offset Set"(w350) -> ()
        n182 = local write "Amplitude Set"(w349) -> ()
      }
      event #10 {
        n183 = event-data() -> ()  [unwired: 7 out]
        n184 = local read "Start Freq. Set"() -> (w362:dbl[unit])
        n185 = local read "Stop Freq. Set"() -> (w361:dbl[unit])
        n186 = call-poly "To Center and Span.vi"("stop"=w361, "start"=w362) -> ("span"=w359:dbl[unit], "center"=w360:dbl[unit])  [unwired: 4 out]
        n187 = local write "Center Freq. Set"(w360) -> ()
        n188 = local write "Freq. Span Set"(w359) -> ()
      }
      event #11 {
        n189 = event-data() -> ()  [unwired: 7 out]
        n190 = local read "Center Freq. Set"() -> (w368:dbl[unit])
        n191 = local read "Freq. Span Set"() -> (w367:dbl[unit])
        n192 = call-poly "To Start and Stop.vi"("span"=w367, "center"=w368) -> ("stop"=w365:dbl[unit], "start"=w366:dbl[unit])  [unwired: 4 out]
        n193 = local write "Start Freq. Set"(w366) -> ()
        n194 = local write "Stop Freq. Set"(w365) -> ()
      }
    }
  }
  n195 = call <vilib>:"Simple Error Handler.vi"("error in (no error)"=w5) -> ("error out"=w4:errorcluster)  [unwired: 1 in, 7 out]
  n196 = call-dynamic "_Destroy.vi"("error in (no error)"=w4, "Instrument in"=w1) -> ("error out"=→"error out":errorcluster)  [unwired: 9 out]
